vi "RTS Get Test State.vi"(10 "TCP Data":string[][](array[string]), 11 "Index of Recording Column":i32) -> (0 "TDMS Locations":path[](array[path]), 1 "Point Locations":path[](array[path]), 2 "Save States":bool[](array[boolean]), 3 "Current Status":string[](array[string]))   [LabVIEW 2016]
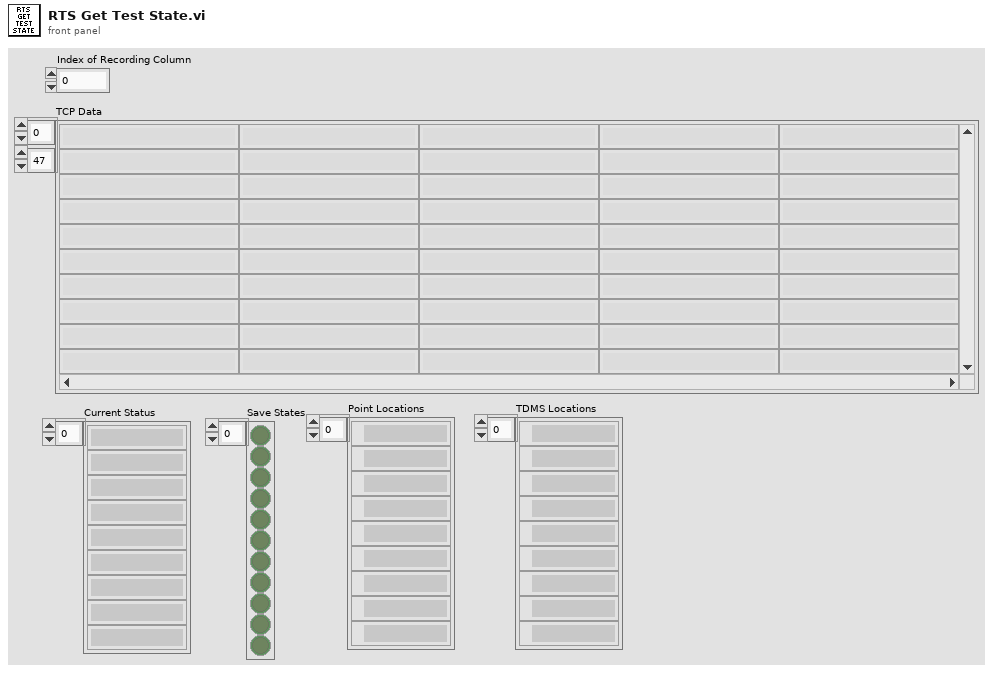
[diagram p1: front panel]
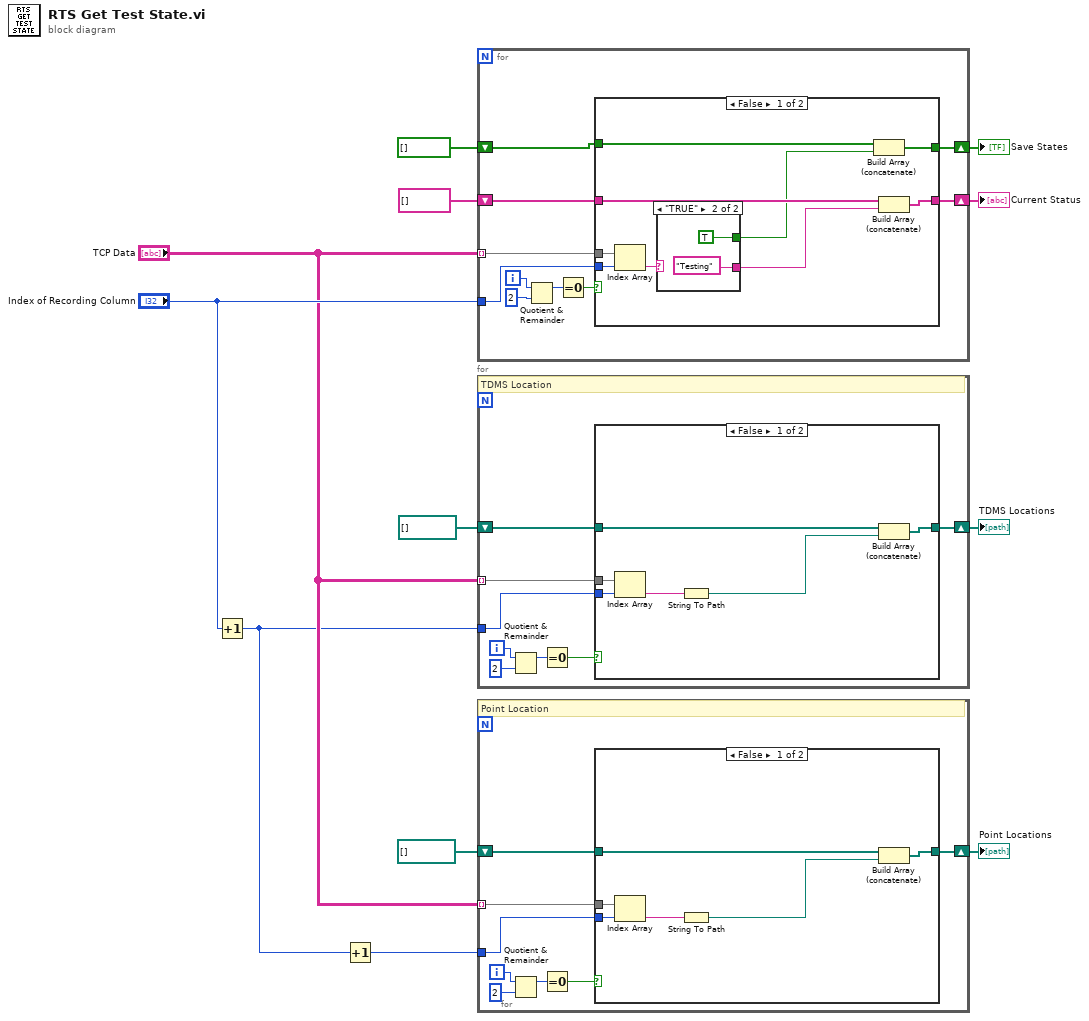
[diagram p0: block diagram]
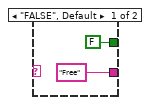
[diagram p4: hidden frame]
diagram:
  n1 = Increment(x="Index of Recording Column") -> (x+1=w2:i32)
  n2 = Increment(x=w2) -> (x+1=w1:i32)
  n3 = for {
    tunnel: "TCP Data" -> [w18] mode=indexing
    tunnel: "Index of Recording Column" -> [w17]
    shift-right: [w15] -> w12
    shift-left: string[] [] -> [w16]
    shift-right: [w13] -> w9
    shift-left: bool[] [] -> [w14]
    i -> [w22]
    n4 = Quotient & Remainder(x=w22, y=2) -> (x-y*floor(x/y)=w20:i32)  [unwired: 1 out]
    n5 = Equal To 0?(x=w20) -> (x = 0?=w19:bool)
    n6 = case shown="False" w19 {
      tunnel: w18 -> [w31 _]
      tunnel: w17 -> [w30 _]
      tunnel: w16 -> [w29 w37]
      tunnel: [w28 w37] -> w15
      tunnel: w14 -> [w25 w36]
      tunnel: [w23 w36] -> w13
      frame False {
        n7 = Index Array(array=w31, index=w30) -> (element=w27:string)
        n8 = case shown="\"TRUE\"" w27 {
          tunnel: ["Free" "Testing"] -> w26
          tunnel: [FALSE TRUE] -> w24
          frame "FALSE", Default {
          }
          frame "TRUE" {
          }
        }
        n9 = Build Array (concatenate)(w25, w24) -> (w23:bool[])
        n10 = Build Array (concatenate)(w29, w26) -> (w28:string[])
      }
      frame True {
      }
    }
  }
  "Current Status" <- w12
  "Save States" <- w9
  n11 = for {
    tunnel: "TCP Data" -> [w41] mode=indexing
    tunnel: w2 -> [w40]
    shift-right: [w38] -> w5
    shift-left: path[] [] -> [w39]
    i -> [w45]
    # "TDMS Location"
    n12 = Quotient & Remainder(x=w45, y=2) -> (x-y*floor(x/y)=w43:i32)  [unwired: 1 out]
    n13 = Equal To 0?(x=w43) -> (x = 0?=w42:bool)
    n14 = case shown="False" w42 {
      tunnel: w41 -> [w51 _]
      tunnel: w40 -> [w50 _]
      tunnel: w39 -> [w49 w52]
      tunnel: [w48 w52] -> w38
      frame False {
        n15 = Index Array(array=w51, index=w50) -> (element=w47:string)
        n16 = String To Path(string=w47) -> (path=w46:path)
        n17 = Build Array (concatenate)(w49, w46) -> (w48:path[])
      }
      frame True {
      }
    }
  }
  "TDMS Locations" <- w5
  n18 = for {
    tunnel: "TCP Data" -> [w56] mode=indexing
    tunnel: w1 -> [w55]
    shift-right: [w53] -> w4
    shift-left: path[] [] -> [w54]
    i -> [w60]
    # "Point Location"
    n19 = Quotient & Remainder(x=w60, y=2) -> (x-y*floor(x/y)=w58:i32)  [unwired: 1 out]
    n20 = Equal To 0?(x=w58) -> (x = 0?=w57:bool)
    n21 = case shown="False" w57 {
      tunnel: w56 -> [w66 _]
      tunnel: w55 -> [w65 _]
      tunnel: w54 -> [w64 w67]
      tunnel: [w63 w67] -> w53
      frame False {
        n22 = Index Array(array=w66, index=w65) -> (element=w62:string)
        n23 = String To Path(string=w62) -> (path=w61:path)
        n24 = Build Array (concatenate)(w64, w61) -> (w63:path[])
      }
      frame True {
      }
    }
  }
  "Point Locations" <- w4
